vi "Test System.vi"() -> ()   [LabVIEW 2014]
uses:
  CAN Communication/PAS/PAS.lvclass
  Common/Buffers/Snapshot/Snapshot.lvclass
  CAN Communication/Peltier/Peltier.lvclass
  CAN Communication/Peltier/Typedefs/Peltier Temperature Sensors.ctl
  CAN Communication/PAS/Typedefs/Valves.ctl
panel:
  out "Status":string
  out "Temp":dbl caption="H2 Temp C" format="%#.2g"
  out "PPM":dbl caption="H2 PPM" format="%#.2g"
  in  "H2":bool
  out "Gas Board Errors":errorcluster
  out "Oil Present?":string
  in  "Oil Pres":bool
  out "Pelt":errorcluster caption="Peltier Board Errors"
  out "TS5":dbl caption="Temp Sensor 5" format="%#.2g"
  out "TS4":dbl caption="Temp Sensor 4" format="%#.2g"
  out "TS3":dbl caption="Temp Sensor 3" format="%#.2g"
  out "TS2":dbl caption="Temp Sensor 2" format="%#.2g"
  out "TS1":dbl caption="Temp Sensor 1" format="%#.2g"
  in  "Pelt":bool
  out "DAQ Errors":errorcluster
  out "Gas Pressure EX (PSI)":dbl format="%#.2g"
  in  "Valves":T1=52 items=["GV1"=33, "GV2"=34, "GV3"=35, "GV4"=36, "GV5"=37, "GV6"=38, "GV7"=39, "GV8"=40, "GV9"=41, "GV10"=42, "GV11"=43, "LV3"=51, "LV4"=52]
  out "Gas Pressure GC (PSI)":dbl format="%#.2g"
  in  "OK Button":bool
  out "Test Pressure (PSI)":dbl format="%#.2g"
  # "On Demand Information"
  # "Pressure Readings"
  # "Gas Board"
  # "Peltier Board"
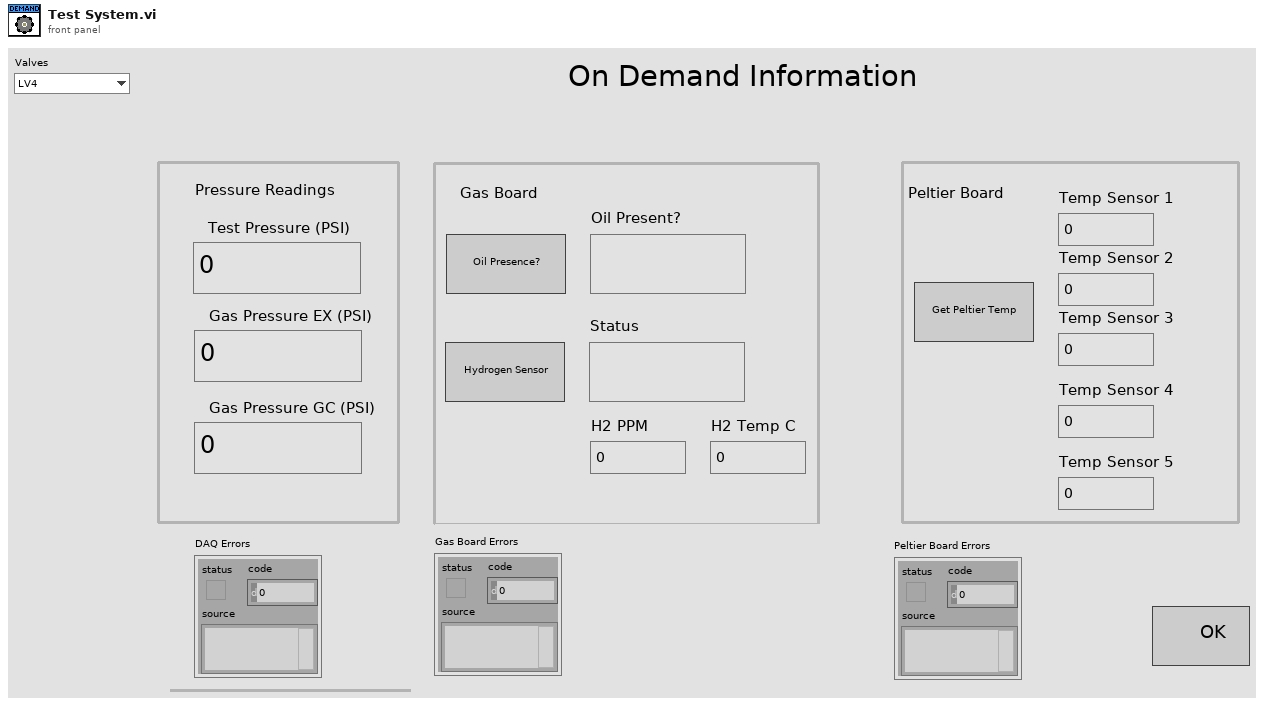
[diagram p1: front panel]
types:
  T1 = typedef "PAS.lvclass/Valves.ctl" = u16
  T2 = typedef "PAS.lvclass/Session Handle.ctl" = refnum<data-value>
  T3 = typedef "Snapshot.lvclass/Session Handle.ctl" = refnum<data-value>
  T4 = typedef "Peltier.lvclass/Peltier Temperature Sensors.ctl" = u16
  T5 = typedef "Peltier.lvclass/Session Handle.ctl" = refnum<data-value>
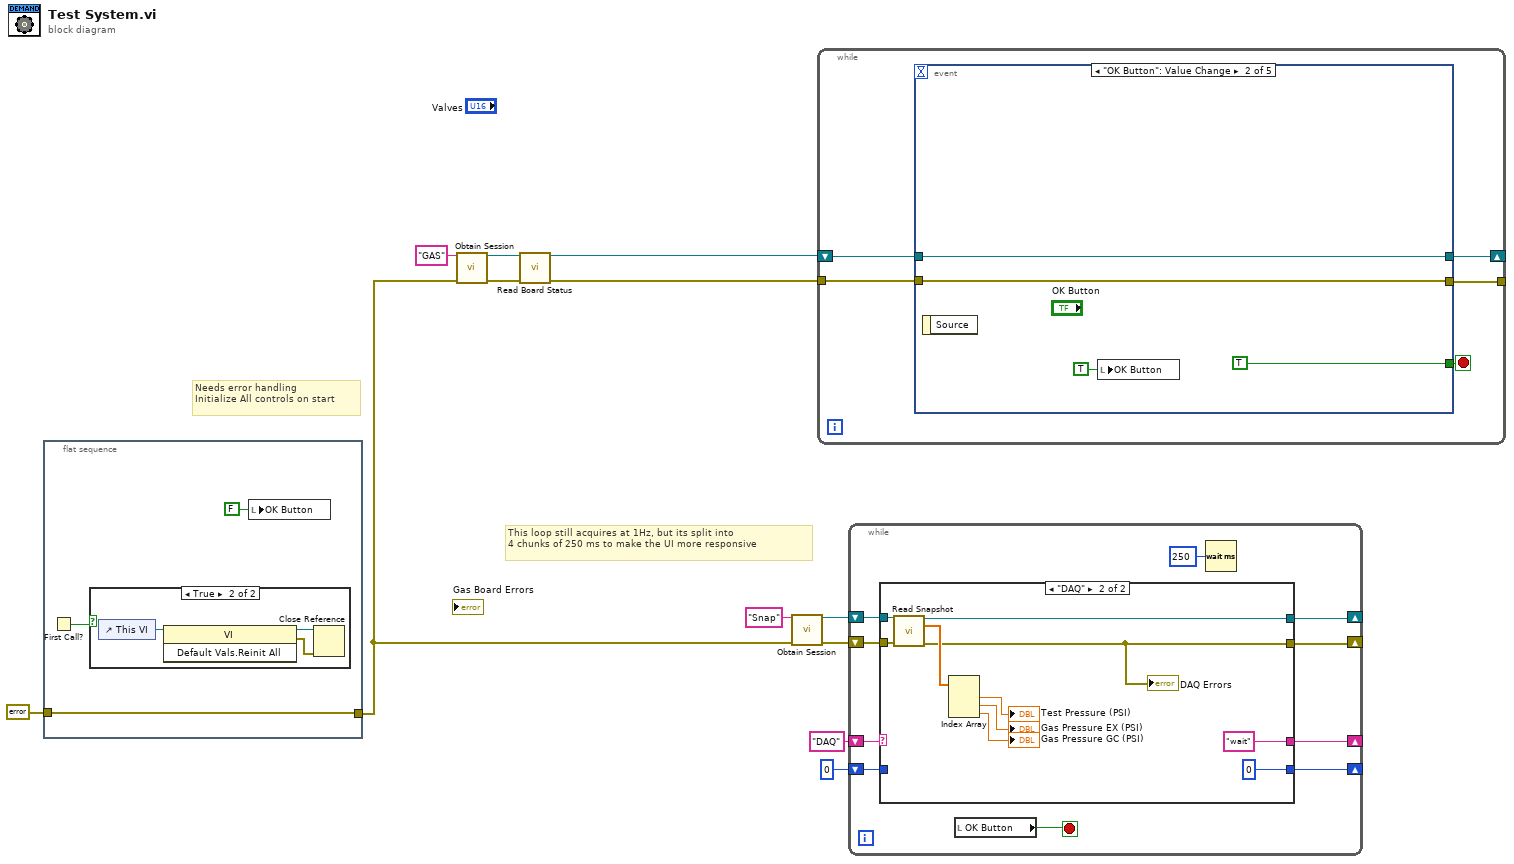
[diagram p0: block diagram]
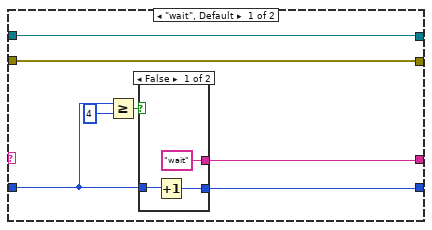
[diagram p2: hidden frame]
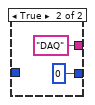
[diagram p3: hidden frame]
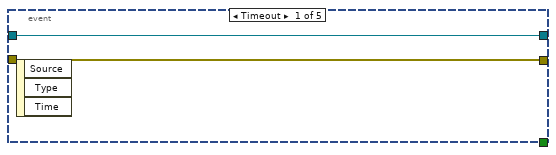
[diagram p5: hidden frame]
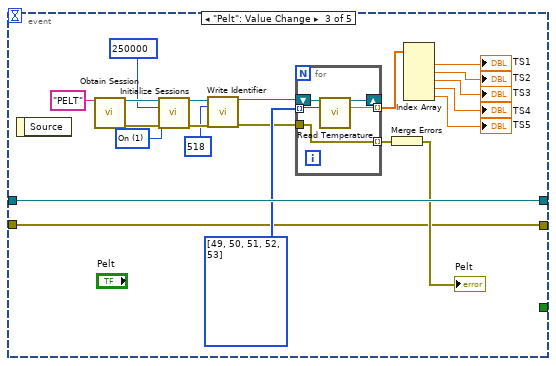
[diagram p6: hidden frame]
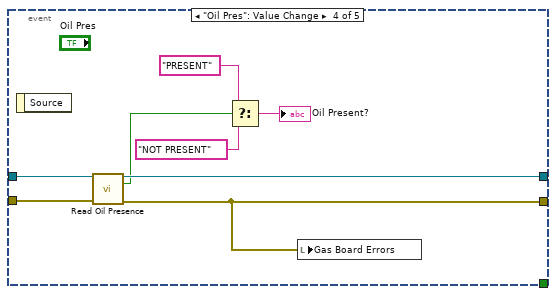
[diagram p7: hidden frame]
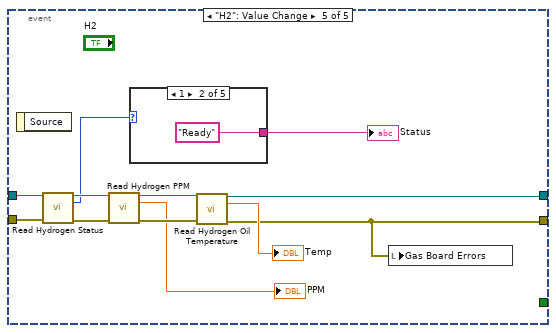
[diagram p8: hidden frame]
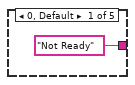
[diagram p9: hidden frame]
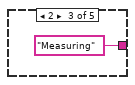
[diagram p10: hidden frame]
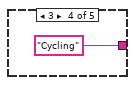
[diagram p11: hidden frame]
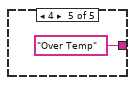
[diagram p12: hidden frame]
diagram:
  # "This loop still acquires at 1Hz, but its split into\n4 chunks of 250 ms to make the UI more responsive"
  # "Needs error handling\nInitialize All controls on start"
  n1 = flat-sequence {
    tunnel: errorcluster {"status"=FALSE, "code"=0, "source"=""} ("error in (no error)") -> [w14]
    tunnel: [w14] -> w1
    frame #0 {
      n2 = First Call?() -> (First Call?: T/F=w13:bool)
      n3 = case shown="True" w13 {
        frame False {
        }
        frame True {
          n4 = control-ref of="This VI"() -> (w18:refnum<vi>)
          n5 = invoke class="VI" method="Default Vals.Reinit All"(reference=w18) -> (reference out=w16:refnum<vi>, error out=w17:errorcluster)  [unwired: 2 in, 1 out]
          n6 = Close Reference(reference=w16, error in (no error)=w17) -> ()  [unwired: 1 out]
        }
      }
      n7 = local write "OK Button"(FALSE ("OK Button")) -> ()
    }
  }
  n8 = call "Obtain Session.vi"("Session  Name ()"="GAS", "error in (no error)"=w1) -> ("Session Handle"=w10:T2, "error out"=w9:errorcluster)  [unwired: 12 in]
  n9 = call "Read Board Status.vi"("Session Handle in"=w10, "error in (no error)"=w9) -> ("Session Handle out"=w8:T2, "error out"=w7:errorcluster)  [unwired: 11 in, 1 out]
  n10 = call "Obtain Session.vi"("Session  Name ()"="Snap", "error in (no error)"=w1) -> ("Session Handle"=w5:T3, "error out"=w4:errorcluster)  [unwired: 12 in]
  n11 = while {
    shift-right: [w21] -> _
    shift-left: w8 -> [w23]
    tunnel: w7 -> [w22]
    tunnel: [w20] -> _
    stop <- w19 stop-if-true
    n12 = event shown="[1] \"OK Button\": Value Change" {
      selector: _ -> [_ _ _ _ _]
      dyn-events: _ -> [_ _ _ _ _]
      timeout: _ -> [_ _ _ _ _]
      tunnel: w23 -> [w25 w29 w50 w62 w74]
      tunnel: w22 -> [w24 w28 w30 w63 w75]
      tunnel: [w25 w29 w50 w61 w68] -> w21
      tunnel: [w24 w28 w30 w56 w64] -> w20
      tunnel: [_ TRUE ("OK Button") _ _ _] -> w19
      event Timeout {
        n13 = event-data() -> ()  [unwired: 1 in, 3 out]
      }
      event "OK Button": Value Change {
        n14 = event-data() -> ()  [unwired: 1 in, 1 out]
        n15 = local write "OK Button"(TRUE ("OK Button")) -> ()
      }
      event "Pelt": Value Change {
        w41 = T4[] [49, 50, 51, 52, 53] items=["PTS1"=49, "PTS2"=50, "PTS3"=51, "PTS4"=52, "PTS5"=53, "PTS6"=54]
        w45 = u32 1 items=["Off", "On"] ("Termination")
        n16 = event-data() -> ()  [unwired: 1 in, 1 out]
        n17 = call "Obtain Session.vi"("Session  Name ()"="PELT") -> ("Session Handle"=w48:T5, "error out"=w47:errorcluster)  [unwired: 13 in]
        n18 = call "Initialize Sessions.vi"("Session Handle"=w48, "Baud Rate"=u32 250000, "Termination"=w45, "error in (no error)"=w47) -> ("Session Handle Out"=w44:T5, "error out"=w43:errorcluster)  [unwired: 10 in]
        n19 = call "Write Identifier.vi"("Session Handle In"=w44, "identifier"=u16 518, "error in (no error)"=w43) -> ("Session Handle Out"=w40:T5, "error out"=w39:errorcluster)  [unwired: 11 in]
        n20 = for {
          shift-right: [w54] -> _
          shift-left: w40 -> [w55]
          tunnel: [w53] -> w38 mode=indexing
          tunnel: w41 -> [w52] mode=indexing
          tunnel: w39 -> [w51]
          tunnel: [w51] -> w37 mode=indexing
          n21 = call "Read Temperature.vi"("Session Handle"=w55, "Pelt Temp Sensors"=w52) -> ("Session Handle Out"=w54:T5, "Temperature"=w53:dbl)  [unwired: 11 in, 1 out]
        }
        n22 = Merge Errors(w37) -> (→"Pelt":errorcluster)
        n23 = Index Array(array=w38) -> (element #1=→"TS1":dbl, element #2=→"TS2":dbl, element #3=→"TS3":dbl, element #4=→"TS4":dbl, element #5=→"TS5":dbl)  [unwired: 5 in]
      }
      event "Oil Pres": Value Change {
        n24 = event-data() -> ()  [unwired: 1 in, 1 out]
        n25 = call "Read Oil Presence.vi"("Session Handle in"=w62, "error in (no error)"=w63) -> ("Session Handle out"=w61:T2, "Present?"=w57:bool, "error out"=w56:errorcluster)  [unwired: 11 in]
        n26 = Select(t="PRESENT", s=w57, f="NOT PRESENT") -> (s? t:f=→"Oil Present?":string)
        n27 = local write "Gas Board Errors"(w56) -> ()
      }
      event "H2": Value Change {
        n28 = event-data() -> ()  [unwired: 1 in, 1 out]
        n29 = call "Read Hydrogen Status.vi"("Session Handle in"=w74, "error in (no error)"=w75) -> ("Session Handle out"=w70:T2, "Status"=w65:u16, "error out"=w69:errorcluster)  [unwired: 8 in, 3 out]
        n30 = call "Read Hydrogen PPM.vi"("Session Handle in"=w70, "error in (no error)"=w69) -> ("Session Handle out"=w72:T2, "H2 PPM"=→"PPM":dbl, "error out"=w71:errorcluster)  [unwired: 10 in, 1 out]
        n31 = case shown="1" w65 {
          tunnel: ["Not Ready" "Ready" "Measuring" "Cycling" "Over Temp"] -> w73
          frame 0, Default {
          }
          frame 1 {
          }
          frame 2 {
          }
          frame 3 {
          }
          frame 4 {
          }
        }
        "Status" <- w73
        n32 = call "Read Hydrogen Oil Temperature.vi"("Session Handle in"=w72, "error in (no error)"=w71) -> ("Session Handle out"=w68:T2, "H2 Temp"=→"Temp":dbl, "error out"=w64:errorcluster)  [unwired: 10 in, 1 out]
        n33 = local write "Gas Board Errors"(w64) -> ()
      }
    }
  }
  n34 = while {
    shift-right: [w87] -> _
    shift-left: w5 -> [w88]
    shift-right: [w86] -> _
    shift-left: w4 -> [w89]
    shift-right: [w84] -> _
    shift-left: "DAQ" -> [w85]
    shift-right: [w83] -> _
    shift-left: 0 -> [w82]
    stop <- w90 stop-if-true
    n35 = case shown="\"DAQ\"" w85 {
      tunnel: w89 -> [w96 w112]
      tunnel: w88 -> [w97 w111]
      tunnel: [w97 w110] -> w87
      tunnel: [w96 w103] -> w86
      tunnel: [w91 "wait"] -> w84
      tunnel: [w92 0] -> w83
      tunnel: w82 -> [w93 _]
      frame "wait", Default {
        n36 = Greater Or Equal?(x=w93, y=4) -> (x >= y?=w94:bool)
        n37 = case shown="False" w94 {
          tunnel: w93 -> [w100 _]
          tunnel: [w99 0] -> w92
          tunnel: ["wait" "DAQ"] -> w91
          frame False {
            n38 = Increment(x=w100) -> (x+1=w99:i32)
          }
          frame True {
          }
        }
      }
      frame "DAQ" {
        n39 = call "Read Snapshot.vi"("Session Handle in"=w111, "error in (no error)"=w112) -> ("Session Handle out"=w110:T3, "Buffer"=w109:dbl[], "error out"=w103:errorcluster)  [unwired: 11 in]
        "DAQ Errors" <- w103
        n40 = Index Array(array=w109) -> (element #1=→"Test Pressure (PSI)":dbl, element #2=→"Gas Pressure EX (PSI)":dbl, element #3=→"Gas Pressure GC (PSI)":dbl)  [unwired: 3 in]
      }
    }
    n41 = local read "OK Button"() -> (w90:bool)
    n42 = Wait (ms)(milliseconds to wait=u32 250) -> ()  [unwired: 1 out]
  }
